vi "FMDLKeithley2450InitiateImmediateReadDataClearBuffer.vi"(7 "error in (no error)":errorcluster, 8 "Timeout (10000 ms)":u32=10000, 9 "Buffer Name (defbuffer1)":string="defbuffer1", 10 "VISA resource name":refnum<visa-resource-name>) -> (0 "error out":errorcluster, 1 "StDev":dbl, 2 "Mean":dbl, 3 "VISA resource name out":refnum<visa-resource-name>, 4 "PkToPk":dbl, 5 "Minimum":dbl, 6 "Maximum":dbl)   [LabVIEW 2018]
uses:
  <instrlib>/Keithley 2450/Keithley 2450.lvlib
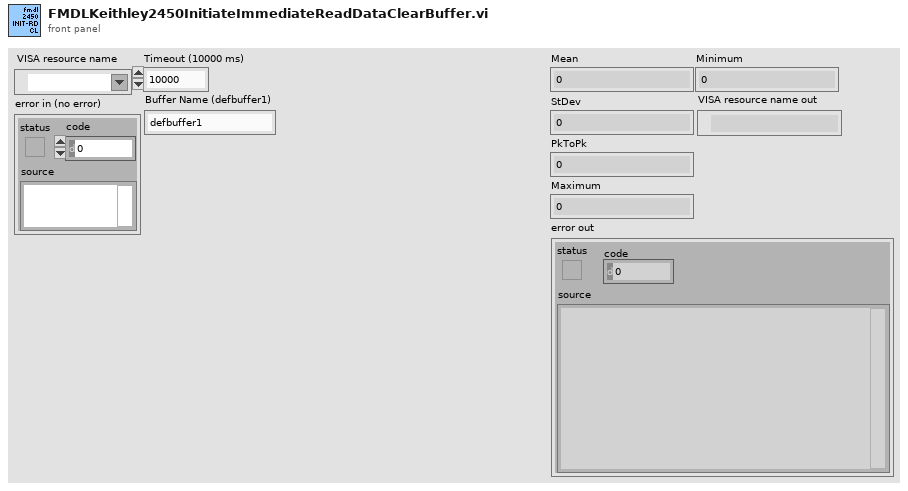
[diagram p1: front panel]
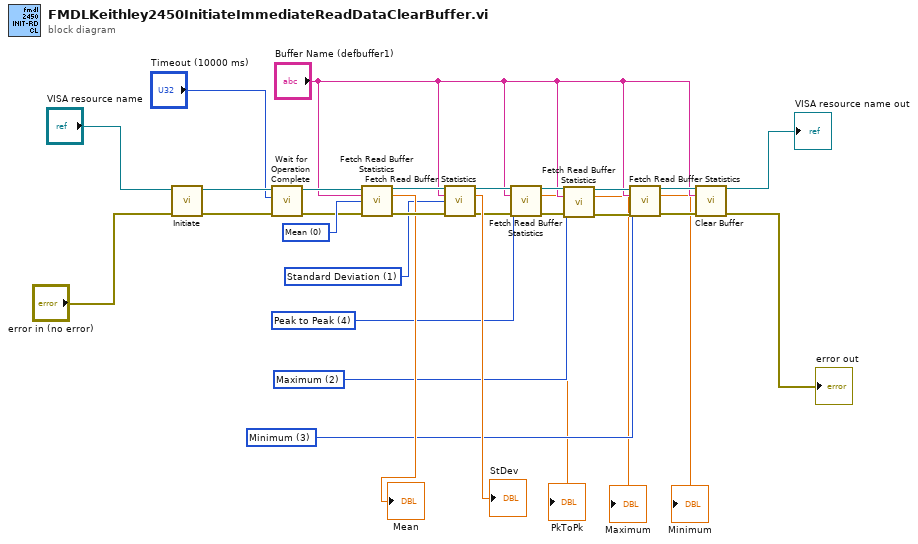
[diagram p0: block diagram]
diagram:
  w7 = u16 3 items=["Mean", "Standard Deviation", "Maximum", "Minimum", "Peak to Peak"] ("Statistical Operation (0: Mean)")
  w8 = u16 2 items=["Mean", "Standard Deviation", "Maximum", "Minimum", "Peak to Peak"] ("Statistical Operation (0: Mean)")
  w16 = u16 4 items=["Mean", "Standard Deviation", "Maximum", "Minimum", "Peak to Peak"] ("Statistical Operation (0: Mean)")
  w6 = u16 1 items=["Mean", "Standard Deviation", "Maximum", "Minimum", "Peak to Peak"] ("Statistical Operation (0: Mean)")
  w30 = u16 0 items=["Mean", "Standard Deviation", "Maximum", "Minimum", "Peak to Peak"] ("Statistical Operation (0: Mean)")
  n1 = call <instrlib>:"Initiate.vi"("error in (no error)"="error in (no error)", "VISA resource name"="VISA resource name") -> ("error out"=w27:errorcluster, "VISA resource name out"=w29:refnum<visa-resource-name>)  [unwired: 8 in]
  n2 = call <instrlib>:"Wait for Operation Complete.vi"("error in (no error)"=w27, "Timeout (10000 ms)"="Timeout (10000 ms)", "VISA resource name"=w29) -> ("error out"=w26:errorcluster, "VISA resource name out"=w28:refnum<visa-resource-name>)  [unwired: 7 in]
  n3 = call <instrlib>:"Fetch Read Buffer Statistics.vi"("VISA resource name"=w28, "Buffer Name (defbuffer1)"="Buffer Name (defbuffer1)", "Statistical Operation (0: Mean)"=w30, "error in (no error)"=w26) -> ("VISA resource name out"=w22:refnum<visa-resource-name>, "Data Out"=→"Mean":dbl, "error out"=w21:errorcluster)  [unwired: 9 in]
  n4 = call <instrlib>:"Fetch Read Buffer Statistics.vi"("VISA resource name"=w22, "Buffer Name (defbuffer1)"="Buffer Name (defbuffer1)", "Statistical Operation (0: Mean)"=w6, "error in (no error)"=w21) -> ("VISA resource name out"=w18:refnum<visa-resource-name>, "Data Out"=→"StDev":dbl, "error out"=w17:errorcluster)  [unwired: 9 in]
  n5 = call <instrlib>:"Fetch Read Buffer Statistics.vi"("VISA resource name"=w18, "Buffer Name (defbuffer1)"="Buffer Name (defbuffer1)", "Statistical Operation (0: Mean)"=w16, "error in (no error)"=w17) -> ("VISA resource name out"=w15:refnum<visa-resource-name>, "Data Out"=→"PkToPk":dbl, "error out"=w14:errorcluster)  [unwired: 9 in]
  n6 = call <instrlib>:"Fetch Read Buffer Statistics.vi"("VISA resource name"=w15, "Buffer Name (defbuffer1)"="Buffer Name (defbuffer1)", "Statistical Operation (0: Mean)"=w8, "error in (no error)"=w14) -> ("VISA resource name out"=w13:refnum<visa-resource-name>, "Data Out"=→"Maximum":dbl, "error out"=w12:errorcluster)  [unwired: 9 in]
  n7 = call <instrlib>:"Fetch Read Buffer Statistics.vi"("VISA resource name"=w13, "Buffer Name (defbuffer1)"="Buffer Name (defbuffer1)", "Statistical Operation (0: Mean)"=w7, "error in (no error)"=w12) -> ("VISA resource name out"=w11:refnum<visa-resource-name>, "Data Out"=→"Minimum":dbl, "error out"=w10:errorcluster)  [unwired: 9 in]
  n8 = call <instrlib>:"Clear Buffer.vi"("VISA resource name"=w11, "Buffer Name (defbuffer1)"="Buffer Name (defbuffer1)", "error in (no error)"=w10) -> ("VISA resource name out"=→"VISA resource name out":refnum<visa-resource-name>, "error out"=→"error out":errorcluster)  [unwired: 11 in]
